vi "VCS Get Ssi Abs Encoder Parameter.vi"(6 "error in (no error)":errorcluster, 9 "axis in":cluster{"keyHandle":u32, "nodeId":u16}={"keyHandle"=0, "nodeId"=1}) -> (0 "error out":errorcluster, 2 "SSI encoder parameter":T1, 3 "axis out":cluster{"keyHandle":u32, "nodeId":u16}={"keyHandle"=0, "nodeId"=1})   [LabVIEW 2010]
doc: "With function <B>VCS_GetSsiAbsEncoderParameter</B> it is possible to read all parameters from SSI absolute encoder."
uses:
  Resources/EposCmd.dll
  Resources/EposCmd64.dll
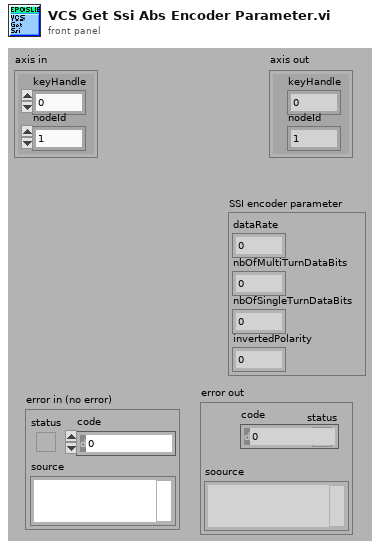
[diagram p1: front panel]
types:
  T1 = cluster{"dataRate":u16, "nbOfMultiTurnDataBits":u16, "nbOfSingleTurnDataBits":u16, "invertedPolarity":i32}
  T2 = cluster{"pDataRate":u16, "pNbOfMultiTurnDataBits":u16, "pNbOfSingleTurnDataBits":u16, "pInvertedPolarity":i32}
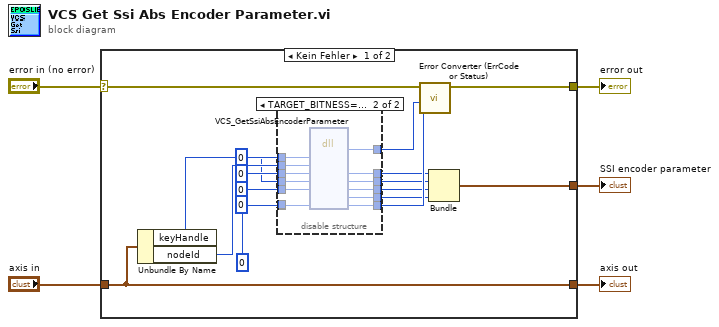
[diagram p0: block diagram]
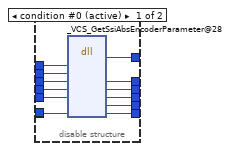
[diagram p2: hidden frame]
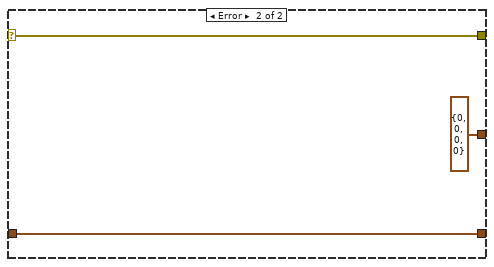
[diagram p3: hidden frame]
diagram:
  n1 = case shown="Kein Fehler" "error in (no error)" {
    selector: "error in (no error)" -> [w20 w50]
    tunnel: "axis in" -> [w22 w51]
    tunnel: [w22 w51] -> w4
    tunnel: [w21 w50] -> w3
    tunnel: [w10 T2 {"pDataRate"=0, "pNbOfMultiTurnDataBits"=0, "pNbOfSingleTurnDataBits"=0, "pInvertedPolarity"=0}] -> w1
    frame No Error {
      n2 = Unbundle By Name(w22) -> ("keyHandle"=w19:u32, "nodeId"=w18:u16)
      n3 = disable-structure shown="TARGET_BITNESS==64" {
        disable-tunnel: w19 -> [w35 w48]
        disable-tunnel: w18 -> [w34 w47]
        disable-tunnel: u32 0 ("pErrorCode") -> [w33 w46]
        disable-tunnel: [w32 w45] -> w16
        disable-tunnel: [w31 w44] -> w15
        disable-tunnel: [w30 w43] -> w14
        disable-tunnel: [w29 w42] -> w13
        disable-tunnel: [w28 w41] -> w12
        disable-tunnel: [w27 w40] -> w11
        disable-tunnel: u16 0 ("pDataRate") -> [w26 w39]
        disable-tunnel: u16 0 ("pNbOfMultiTurnDataBits") -> [w25 w38]
        disable-tunnel: u16 0 ("pNbOfSingleTurnDataBits") -> [w24 w37]
        disable-tunnel: 0 ("pInvertedPolarity") -> [w23 w36]
        frame condition #0 (active) {
          n4 = dll-call lib="C:/Sources/LabVIEW/maxon EPOS/Resources/EposCmd.*" fn="_VCS_GetSsiAbsEncoderParameter@28"("KeyHandle"=w35, "NodeId"=w34, "pDataRate"=w26, "pNbOfMultiTurnDataBits"=w25, "pNbOfSingleTurnDataBits"=w24, "pInvertedPolarity"=w23, "pErrorCode"=w33) -> (w31:i32, "pDataRate"=w30:u16, "pNbOfMultiTurnDataBits"=w29:u16, "pNbOfSingleTurnDataBits"=w28:u16, "pInvertedPolarity"=w27:i32, "pErrorCode"=w32:u32)  [unwired: 5 in, 2 out]
        }
        frame condition #1 {
          n5 = dll-call lib="C:/Sources/LabVIEW/maxon EPOS/Resources/EposCmd64.dll" fn="VCS_GetSsiAbsEncoderParameter" ("EposCmd.dll:_VCS_GetSsiAbsEncoderParameter@28")("KeyHandle"=w48, "NodeId"=w47, "pDataRate"=w39, "pNbOfMultiTurnDataBits"=w38, "pNbOfSingleTurnDataBits"=w37, "pInvertedPolarity"=w36, "pErrorCode"=w46) -> ("Rückgabetyp"=w44:i32, "pDataRate"=w43:u16, "pNbOfMultiTurnDataBits"=w42:u16, "pNbOfSingleTurnDataBits"=w41:u16, "pInvertedPolarity"=w40:i32, "pErrorCode"=w45:u32)  [unwired: 5 in, 2 out]
        }
      }
      n6 = call "Error Converter (ErrCode or Status).vi"("error code"=w16, "return type"=w15, "error in (no error)"=w20) -> ("error out"=w21:errorcluster)  [unwired: 7 in]
      n7 = Bundle("pDataRate"=w14, "pNbOfMultiTurnDataBits"=w13, "pNbOfSingleTurnDataBits"=w12, "pInvertedPolarity"=w11) -> (w10:T2)  [unwired: 1 in]
    }
    frame Error {
    }
  }
  "error out" <- w3
  "axis out" <- w4
  "SSI encoder parameter" <- w1
